vi "prefixTreeDelimiter.get.vi"(8 "error in (no error)":errorcluster, 11 "channelConfig in":refnum<class "channelConfig.lvclass">) -> (0 "error out":errorcluster, 2 "prefixTreeDelimiter":string, 3 "channelConfig out":refnum<class "channelConfig.lvclass">)   [LabVIEW 2020, in "nominal types.lvlib" / "channelConfig.lvclass"]
uses:
  channelConfig.lvclass
  channelConfig.lvclass/channelConfig.ctl
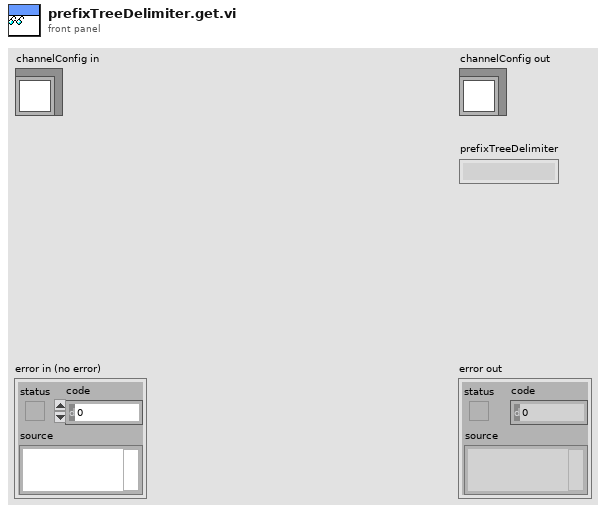
[diagram p1: front panel]
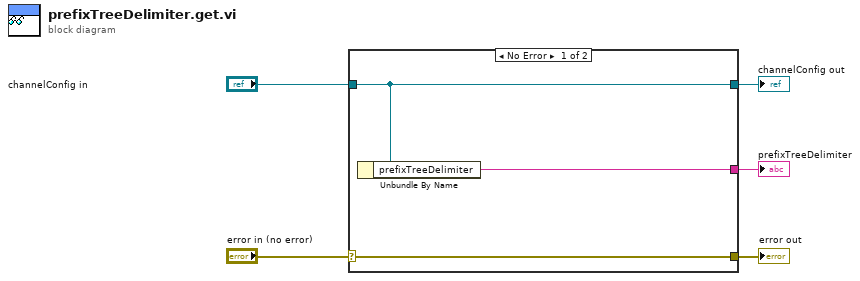
[diagram p0: block diagram]
diagram:
  n1 = case shown="No Error" "error in (no error)" {
    selector: "error in (no error)" -> [w8 w9]
    tunnel: [w8 w9] -> w4
    tunnel: [w7 w10] -> w2
    tunnel: "channelConfig in" -> [w7 w10]
    tunnel: [w6 _] -> w1
    frame No Error {
      n2 = Unbundle By Name(w7) -> ("prefixTreeDelimiter"=w6:string)
    }
    frame Error {
    }
  }
  "error out" <- w4
  "channelConfig out" <- w2
  "prefixTreeDelimiter" <- w1
